vi "Load All Values and Start FPGA.vi"(8 "error in":errorcluster, 11 "Resource name":T1="rio://localhost/RIO0") -> (0 "error out":errorcluster, 1 "Sync Guard Data":fxp<+/-,38,12>[](array[numeric])=[888.2284999489784, 399.7682446986437, -617.0920498371124] format="%.9g", 2 "Data Size":u32, 3 "FPGA Refnum out":T2)   [LabVIEW 2020]
doc: "Author: Scott Hannahs <sth@magnet.fsu.edu>\nCopyright 2018 Florida State University, All rights reserved."
uses:
  RT Controls/FPGA SCH Digitizer Ref.ctl
  <vilib>/userDefined/Silver/nirio_resource_slv.ctl
  <vilib>/FPGAPlugInAG/cRIO-9039/niLvFpga_Open_cRIO-9039.vi
  <vilib>/rvi/interface/common/dynamic/niFpgaDynamicAddResources.vi
  <vilib>/FPGAPlugInAG/Dynamic/niLvFpga_Run_Dynamic.vi
  <vilib>/rvi/errors/niLvFpgaAdjustHostInterfaceError.vi
  RT Server Sub VIs/RT Host Globals.vi
  <vilib>/rvi/interface/nirviOpenFPGA/nirviOpenFPGA.xnode
  FPGA Bitfiles/SCHProtection_SCHMPSFPGA_FPGADigitizeandP_n7korhmryUo.lvbitx
  <vilib>/rvi/interface/nirviMethod/nirviMethod.xnode
  <vilib>/rvi/interface/nirviReadWriteControl/nirviReadWriteControl.xnode
  <vilib>/rvi/interface/Simulation/niFpgaSimulationCallBeginRW.vi
  NiFpgaLv.dll
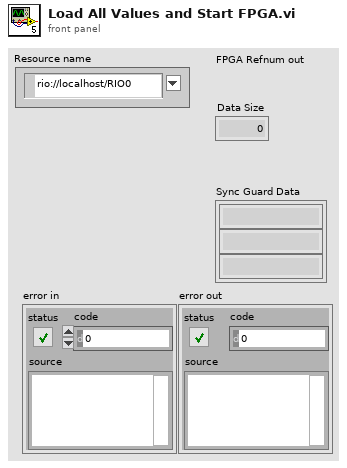
[diagram p1: front panel]
types:
  T1 = typedef "nirio_resource_slv.ctl" = tag
  T2 = typedef "FPGA SCH Digitizer Ref.ctl" = refnum<k20>
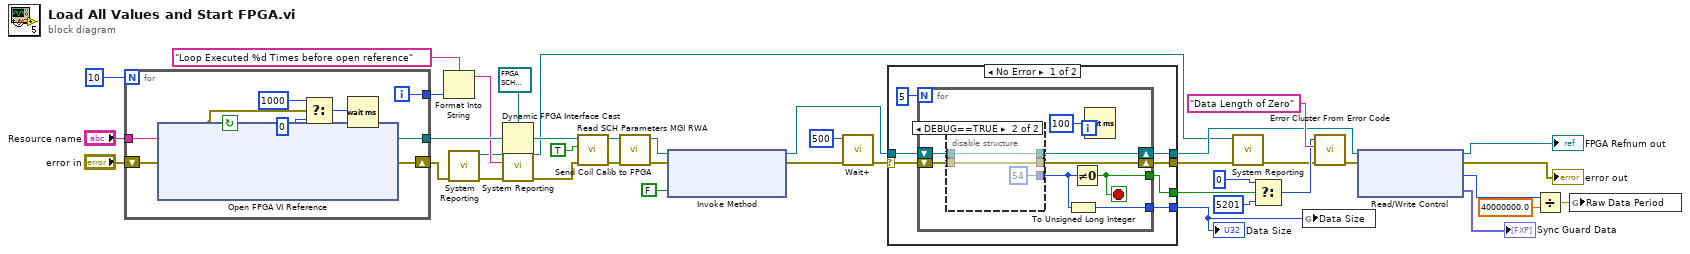
[diagram p0: block diagram]
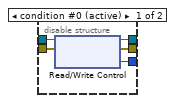
[diagram p2: hidden frame]
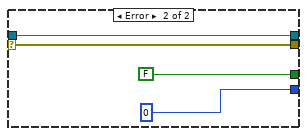
[diagram p3: hidden frame]
diagram:
  n1 = for {
    N: 10 -> [_]
    tunnel: "Resource name" -> [w47]
    tunnel: [w46] -> w22
    shift-right: [w43] -> w11
    shift-left: "error in" -> [w48]
    tunnel: [w41] -> w15
    i -> [w41]
    stop <- w43 continue-if-true
    n2 = xnode "Open FPGA VI Reference"("error in"=w48, "resource name"=w47) -> ("FPGA VI Reference Out"=w46:refnum<k20>, "error out"=w43:errorcluster)
    n3 = Select(t=u32 1000, s=w43, f=u32 0 ("milliseconds to wait")) -> (s? t:f=w45:u32)
    n4 = Wait (ms)(milliseconds to wait=w45) -> ()  [unwired: 1 out]
  }
  n5 = Format Into String(format string="Loop Executed %d Times before open reference", w15) -> (resulting string=w9:string)  [unwired: 2 in, 1 out]
  n6 = call "System Reporting.vi"("Error In"=w11) -> ("Error Out"=w10:errorcluster, "Byte Stream File out"=w8:refnum<file>)  [unwired: 9 in]
  n7 = Dynamic FPGA Interface Cast(Session In=T2 refnum ("FPGA Refnum out"), Type=w22) -> (Session Out=w14:T2)
  n8 = call "System Reporting.vi"("Error In"=w10, "String"=w9, "Byte Stream File in"=w8) -> ("Error Out"=w7:errorcluster, "Byte Stream File out"=w3:refnum<file>)  [unwired: 7 in]
  n9 = call "Read SCH Parameters MGI RWA.vi"("error in (no error)"=w7, "Done"=TRUE, "FPGA Refnum in"=w14) -> ("error out"=w30:errorcluster, "Refnum out"=w21:T2)  [unwired: 7 in]
  n10 = call "Send Coil Calib to FPGA.vi"("error in (no error)"=w30, "Refnum in"=w21) -> ("error out"=w39:errorcluster, "Refnum out"=w20:T2)  [unwired: 7 in, 1 out]
  n11 = xnode "Invoke Method"("FPGA VI Reference In"=w20, "error in"=w39, "Wait Until Done (F)"=FALSE) -> ("FPGA VI Reference Out"=w19:T2, "error out"=w33:errorcluster)
  n12 = call "Wait+.vi"("Error In"=w33, "milliseconds to wait"=u32 500) -> ("Error Out"=w2:errorcluster)  [unwired: 4 in, 1 out]
  n13 = case shown="No Error" w2 {
    selector: w2 -> [w49 w72]
    tunnel: [w54 w72] -> w6
    tunnel: [w53 FALSE] -> w37
    tunnel: w19 -> [w52 w75]
    tunnel: [w51 w75] -> w18
    tunnel: [w50 0 ("Data Size")] -> w23
    frame No Error {
      n14 = for {
        N: 5 -> [_]
        tunnel: [w56] -> w50
        shift-right: [w58] -> w54
        shift-left: w49 -> [w59]
        shift-right: [w60] -> w51
        shift-left: w52 -> [w61]
        tunnel: [w62] -> w53
        stop <- w62 stop-if-true
        n15 = disable-structure shown="DEBUG==TRUE" {
          disable-tunnel: w61 -> [w68 w71]
          disable-tunnel: [w67 w71] -> w60
          disable-tunnel: w59 -> [w66 w70]
          disable-tunnel: [w65 w70] -> w58
          disable-tunnel: [w64 54 ("Data Size")] -> w57
          frame condition #0 (active) {
            n16 = xnode "Read/Write Control"("FPGA VI Reference In"=w68, "error in"=w66) -> ("FPGA VI Reference Out"=w67:T2, "error out"=w65:errorcluster, "Data Size"=w64:i32)
          }
          frame condition #1 {
          }
        }
        n17 = To Unsigned Long Integer(number=w57) -> (unsigned 32bit integer=w56:u32)
        n18 = Not Equal To 0?(x=w57) -> (x != 0?=w62:bool)
        n19 = Wait (ms)(milliseconds to wait=u32 100) -> ()  [unwired: 1 out]
      }
    }
    frame Error {
    }
  }
  "Data Size" <- w23
  n20 = call "System Reporting.vi"("Error In"=w6, "Byte Stream File in"=w3) -> ("Error Out"=w5:errorcluster)  [unwired: 8 in, 1 out]
  n21 = Select(t=0, s=w37, f=5201) -> (s? t:f=w35:i32)
  n22 = global write "RT Host Globals.vi" "Data Size"(w23) -> ()
  n23 = call <vilib>:"Error Cluster From Error Code.vi"("error in (no error)"=w5, "error message (\"\")"="Data Length of Zero" ("error message (\"\")"), "error code (0)"=w35) -> ("error out"=w26:errorcluster)  [unwired: 6 in]
  n24 = xnode "Read/Write Control"("FPGA VI Reference In"=w18, "error in"=w26) -> ("FPGA VI Reference Out"=→"FPGA Refnum out":T2, "error out"=→"error out":errorcluster, "DAQ Cycle Ticks"=w28:u32, "Sync Guard Data"=→"Sync Guard Data":fxp<+/-,38,12>[])
  n25 = Divide(x=w28, y=40000000.0) -> (x/y=w24:dbl)
  n26 = global write "RT Host Globals.vi" "Raw Data Period"(w24) -> ()
